vi "scale UI.vi"() -> ()   [LabVIEW 2013, in "Polynomial Scale editor node.lvclass"]
uses:
  Polynomial Scale editor node.lvclass
  <vilib>/NI/Configuration Framework/Node/NodeRef.ctl
  <vilib>/NI/Configuration Framework/Node/NISE_CEF_Node.lvclass
  <vilib>/NI/AMC/Message Queue.ctl
  <vilib>/NI/AMC/Message.ctl
  <vilib>/NI/Tools/Keyed Array/KeyedArray.ctl
  <vilib>/NI/Configuration Framework/Node/UserEventRef.ctl
  <vilib>/NI/Configuration Framework/Controls/EventCluster.ctl
  <vilib>/NI/Configuration Framework/Node/StopEvent.ctl
  <vilib>/NI/Configuration Framework/Node/RefreshUIEvent.ctl
  <vilib>/NI/Configuration Framework/Node/CacheState.ctl
  <vilib>/NI/Configuration Framework/Node/NodeChangeEvent.ctl
  <vilib>/NI/DCAF Table API/Table Manager/references.ctl
  <vilib>/NI/Tag Bus Data Framework/control module/editor node/channel action event.ctl
  <vilib>/NI/Tag Bus Data Framework/control module/editor node/dialog output action.ctl
  <vilib>/NI/Tag Bus Module Framework/channel/TBM channel.lvclass
  <vilib>/NI/Tag Bus/tag/tag descriptor.lvclass
  <vilib>/NI/Tag Bus Data Framework/Configuration Editor/Classes/Module editor node/module editor node.lvclass
  <vilib>/NI/DCAF Modules/DCAF Scaling/editor node/Scaling editor node.lvclass
  <vilib>/NI/Configuration Framework/NISE_CEF_TreeControl.lvlib
  <vilib>/NI/Tools/Keyed Array/Tools_KeyedArray.lvlib
  <vilib>/NI/AMC/AMC.lvlib
  <vilib>/NI/Tag Bus Data Framework/control module/editor node/control module editor.lvclass
  <vilib>/NI/DCAF Table API/Table Manager/Table Manager.lvclass
panel:
  in  "Coefficients":dbl[](array[numeric])
  in  "node change":T1
  in  "cache state":T2
  in  "refresh UI":T3
  in  "stop event":T4
  in  "user event":T5
  in  "main queue":T6
  in  "node ref":T7
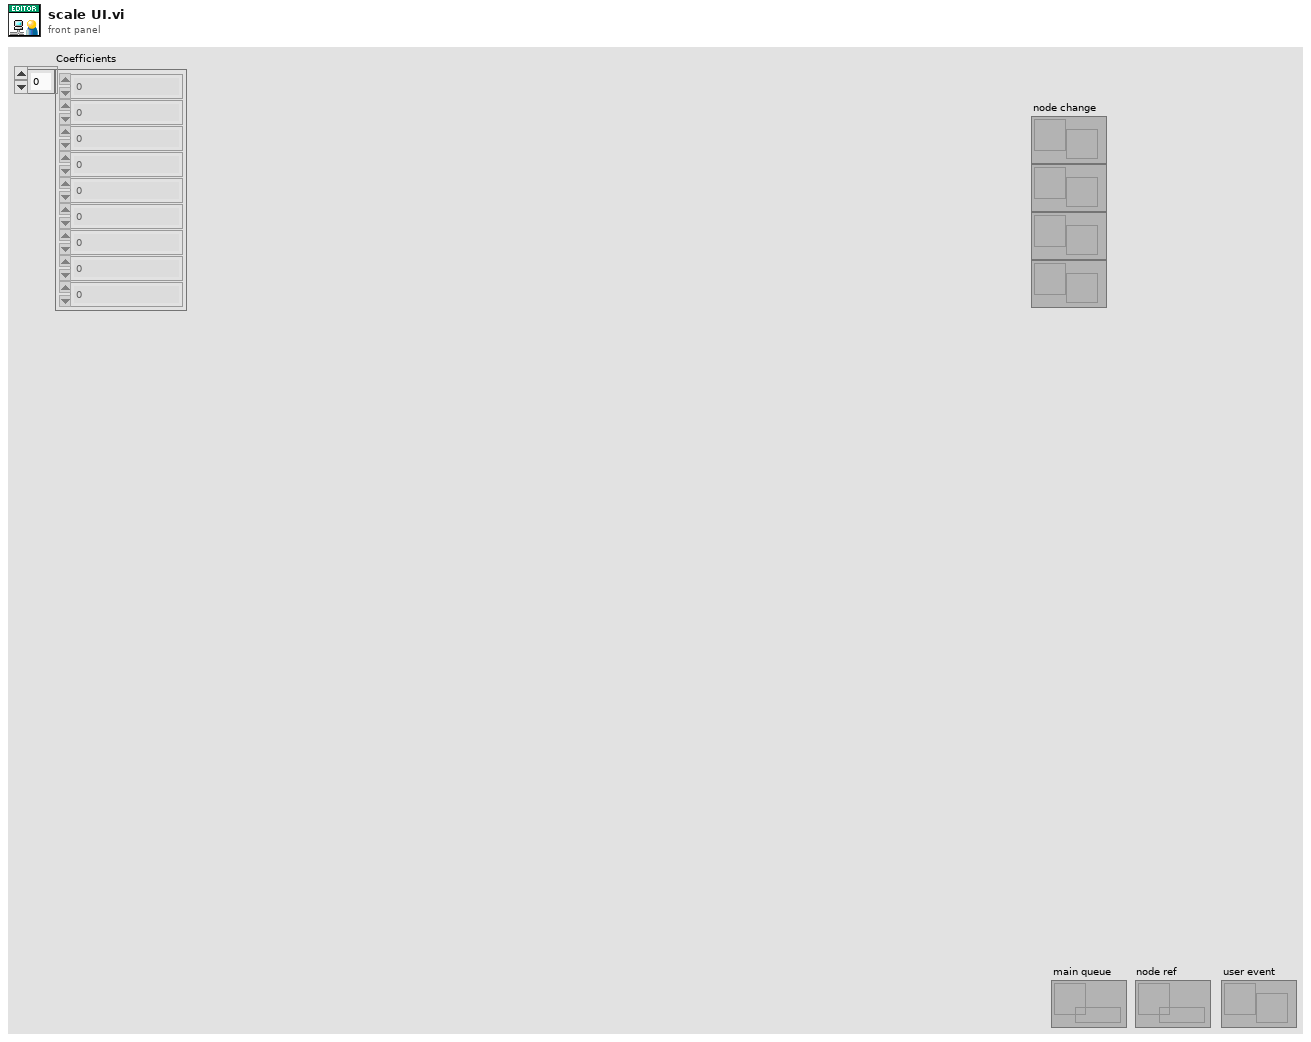
[diagram p1: front panel]
types:
  T1 = typedef "NISE_CEF_Node.lvclass/NodeChangeEvent.ctl" = refnum<user-event>
  T2 = typedef "NISE_CEF_Node.lvclass/CacheState.ctl" = refnum<user-event>
  T3 = typedef "NISE_CEF_Node.lvclass/RefreshUIEvent.ctl" = refnum<user-event>
  T4 = typedef "NISE_CEF_Node.lvclass/StopEvent.ctl" = refnum<user-event>
  T5 = typedef "NISE_CEF_Node.lvclass/UserEventRef.ctl" = refnum<user-event>
  T6 = typedef "AMC.lvlib/Message Queue.ctl" = refnum<queue>
  T7 = typedef "NISE_CEF_Node.lvclass/NodeRef.ctl" = refnum<data-value>
  T8 = typedef "Table Manager.lvlib/Table Manager.lvclass/references.ctl" = cluster{"stop event":T4, "refresh UI":T3, "cache state":T2, "node change":T1, "user event out":refnum<user-event>, "main queue":T6, "user event":T5}
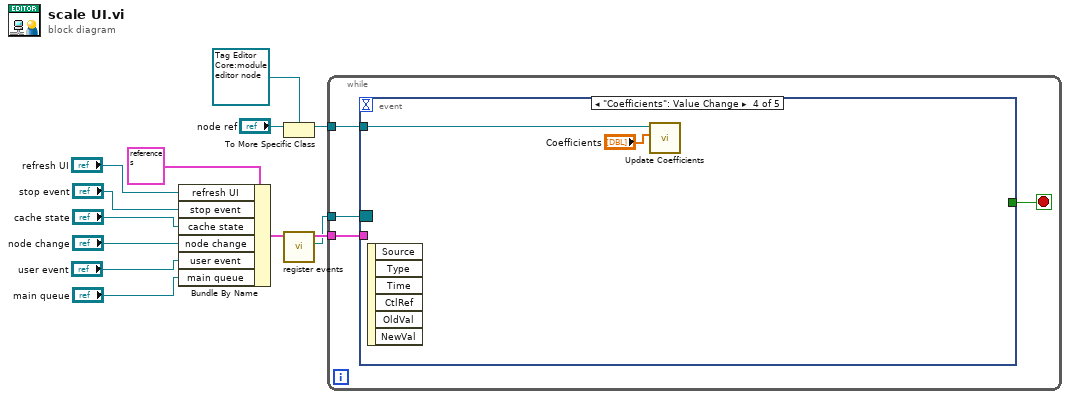
[diagram p0: block diagram]
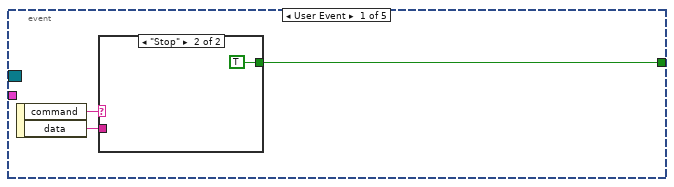
[diagram p2: hidden frame]
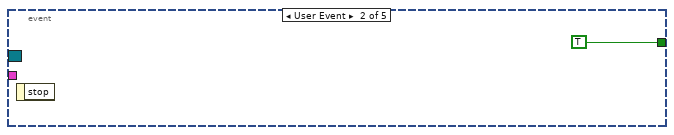
[diagram p4: hidden frame]
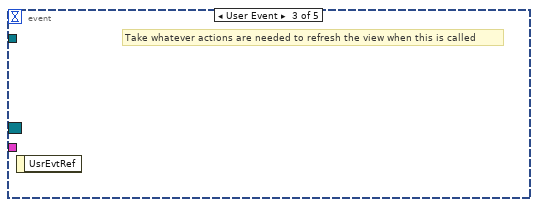
[diagram p5: hidden frame]
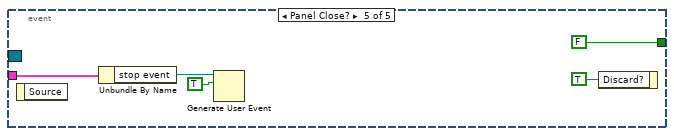
[diagram p6: hidden frame]
diagram:
  n1 = Bundle By Name(cluster=T8 {"stop event"=refnum, "refresh UI"=refnum, "cache state"=refnum, "node change"=refnum, "user event out"=refnum, "main queue"=refnum, "user event"=refnum} ("References in"), "refresh UI"="refresh UI", "stop event"="stop event", "cache state"="cache state", "node change"="node change", "user event"="user event", "main queue"="main queue") -> (w12:T8)
  n2 = To More Specific Class(target class=refnum<data-value> refnum ("data value reference"), reference="node ref") -> (specific class reference=w1:refnum<data-value>)  [unwired: 1 in, 1 out]
  n3 = call <vilib>:"register events.vi"("References"=w12) -> ("Event Registration Refnum"=w4:refnum<event-registration>, "References out"=w5:T8)  [unwired: 8 in, 1 out]
  n4 = while {
    tunnel: w5 -> [w17]
    tunnel: w4 -> [w16]
    tunnel: w1 -> [w14]
    stop <- w15 stop-if-true
    n5 = event shown="[3] \"Coefficients\": Value Change" {
      selector: w16 -> [_ _ _ _ _]
      dyn-events: _ -> [_ _ _ _ _]
      timeout: _ -> [_ _ _ _ _]
      tunnel: [w20 TRUE _ _ FALSE] -> w15
      tunnel: w17 -> [_ _ _ _ w26]
      tunnel: w14 -> [_ _ _ w24 _]
      event User Event {
        n6 = event-data() -> ("command"=w19:string, "data"=w18:string)  [unwired: 1 in]
        n7 = case shown="\"Stop\"" w19 {
          tunnel: [_ TRUE] -> w20
          tunnel: w18 -> [_ _]
          frame Default {
          }
          frame "Stop" {
          }
        }
      }
      event User Event {
        n8 = event-data() -> ()  [unwired: 1 in, 1 out]
      }
      event User Event {
        # "Take whatever actions are needed to refresh the view when this is called"
        n9 = event-data() -> ()  [unwired: 1 in, 1 out]
      }
      event "Coefficients": Value Change {
        n10 = event-data() -> ()  [unwired: 1 in, 6 out]
        n11 = call "Update Coefficients.vi"("coeffs"="Coefficients", "Node Ref"=w24) -> ()  [unwired: 9 in, 1 out]
      }
      event Panel Close? {
        n12 = event-data() -> ()  [unwired: 1 in, 1 out]
        n13 = Unbundle By Name(w26) -> ("stop event"=w25:T4)
        n14 = Generate User Event(user event=w25, event data cluster=TRUE ("event data")) -> ()  [unwired: 2 in, 2 out]
        n15 = event-data("Discard?"=TRUE) -> ()  [unwired: 1 in, 1 out]
      }
    }
  }
